vi "SPD.HV_Bias Test.vi"(5 "Graph":refnum<vi>, 7 "Progress":refnum<vi>, 8 "Error In":errorcluster, 11 "SPD.Stand Ctrl in":T1 {"spdDeviceSession"."hidSPD.Sturtup Values"."HV_bias" format="%#_6p, V"; "spdDeviceSession"."hidSPD.Sturtup Values"."TSet" format="%#_6p, DegC"; "spdDeviceSession"."hidSPD.Controller"."HV_bias" format="%#_6p, V"; "spdDeviceSession"."hidSPD.Controller"."TSet" format="%#_6p, DegC"}) -> (0 "Error Out":errorcluster, 1 "pass":bool, 3 "SPD.Stand Ctrl out":T1 {"spdDeviceSession"."hidSPD.Sturtup Values"."HV_bias" format="%#_6p, V"; "spdDeviceSession"."hidSPD.Sturtup Values"."TSet" format="%#_6p, DegC"; "spdDeviceSession"."hidSPD.Controller"."HV_bias" format="%#_6p, V"; "spdDeviceSession"."hidSPD.Controller"."TSet" format="%#_6p, DegC"})   [LabVIEW 2018]
uses:
  typedefs/SPD.Stand Ctrl.ctl
  Instruments/SPD HID Interface/hidSPDLibForLabView/LibVIs/hidSPD Controls/hidSPD Device Session.ctl
  Instruments/SPD HID Interface/hidSPDLibForLabView/LibVIs/hidSPD Controls/hidSPD Controller.ctl
  Instruments/SPD HID Interface/hidSPDLibForLabView/LibVIs/hidSPD Controls/hidSPD SPD Type.ctl
  Instruments/KC705 DevBoard/typedefs/DevB.Session.ctl
  Instruments/KeySight 53230A/typedefs/FreqC.Session.ctl
  Instruments/KeySight 8164B/KeySight 8164B LAN InstrLib/typedefs/KeySight 8164B control.ctl
  Instruments/LeCroy SDA830/typedefs/LeCroy.Session.ctl
  typedefs/SPD.Events.ctl
  ConfigFile/SPD.Config File ctrl.ctl
  <vilib>/Utility/config.llb/Config Data RefNum.ctl
  typedefs/SPD.Meas Result.ctl
  typedefs/SPD.Queues.ctl
  typedefs/SPD.Stand state.ctl
  SubVIs/Min_Max.ctl
  SubTests/01_HV_Bias Test/SPD.HV_Bias Test Limits.vi
  SubVIs/comparison mode.ctl
  Instruments/KeySight 8164B/KeySight 8164B LAN InstrLib.lvlib
  <vilib>/Utility/config.llb/NI_LVConfig.lvlib
  Instruments/SPD HID Interface/hidSPDLibForLabView/hidSPDLibForLabView.lvlib
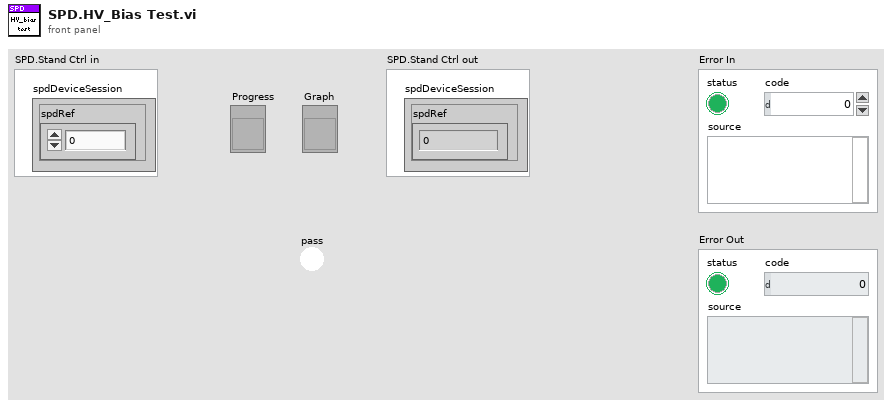
[diagram p1: front panel]
types:
  T1 = typedef "SPD.Stand Ctrl.ctl" = cluster{"spdDeviceSession":T2, "DevBSession":T5, "FreqCSession":T6, "8164BSession":T7, "LeCroySession":T8, "Events":T9, "configFile":T10, "SPD.Result":T12, "SPD.Queues":T13, "Console":refnum<vi>}
  T2 = typedef "hidSPDLibForLabView.lvlib/hidSPD Device Session.ctl" = cluster{"spdRef":u64, "connected":bool, "spdName":string, "hidSPD.Controller":T3, "hidSPD.Sturtup Values":T3, "SPD Type":T4}
  T3 = typedef "hidSPDLibForLabView.lvlib/hidSPD Controller.ctl" = cluster{"TSet":sgl, "HV_bias":sgl, "DDS_stb_code":u16}
  T4 = typedef "hidSPDLibForLabView.lvlib/hidSPD SPD Type.ctl" = enum16{"Free Run", "Gate"}
  T5 = typedef "DevB.Session.ctl" = cluster{"DevBRef":refnum<visa-resource-name>, "connected":bool}
  T6 = typedef "FreqC.Session.ctl" = cluster{"FreqCRef":refnum<visa-resource-name>, "timeout":dbl, "Gate":dbl, "connected":bool}
  T7 = typedef "KeySight 8164B LAN InstrLib.lvlib/KeySight 8164B control.ctl" = cluster{"Connection ID":refnum<k5>, "Connected":bool, "Info":string, "Slots Info":string[]}
  T8 = typedef "LeCroy.Session.ctl" = cluster{"LeCroySession":refnum<visa-resource-name>, "connected":bool}
  T9 = typedef "SPD.Events.ctl" = cluster{"DCRTest":refnum<user-event>, "Stop":refnum<user-event>}
  T10 = typedef "SPD.Config File ctrl.ctl" = cluster{"configFile ref":T11, "configFile path":path, "equipmentFile ref":T11}
  T11 = typedef "NI_LVConfig.lvlib/Config Data RefNum.ctl" = refnum<k1>
  T12 = typedef "SPD.Meas Result.ctl" = cluster{"HV_Bias":dbl[][][], "Stb_code":dbl[], "Temprature":dbl[], "Data":dbl[][][][], "DateTime":string}
  T13 = typedef "SPD.Queues.ctl" = cluster{"state queue":refnum<queue>}
  T14 = typedef "comparison mode.ctl" = enum16{"in range", "bigger then min", "bigger then max", "less then min", "less then max"}
  T15 = typedef "SPD.HV_Bias Test Limits.vi" = cluster{"start value":dbl, "stop value":dbl, "step":dbl, "gate":dbl, "num of tests":dbl, "range":T16, "comparison mode":T14}
  T16 = typedef "Min_Max.ctl" = cluster{"min":dbl, "max":dbl}
  T17 = typedef "SPD.HV_Bias Test Params.vi" = cluster{"FS":i32, "TS":i32, "Step_Quick":dbl, "Stop_Quick":dbl, "Start_Quick":dbl, "Gate_Quick":dbl, "Step_Precise":dbl, "Gate_Precise":dbl, "max":dbl, "min":dbl}
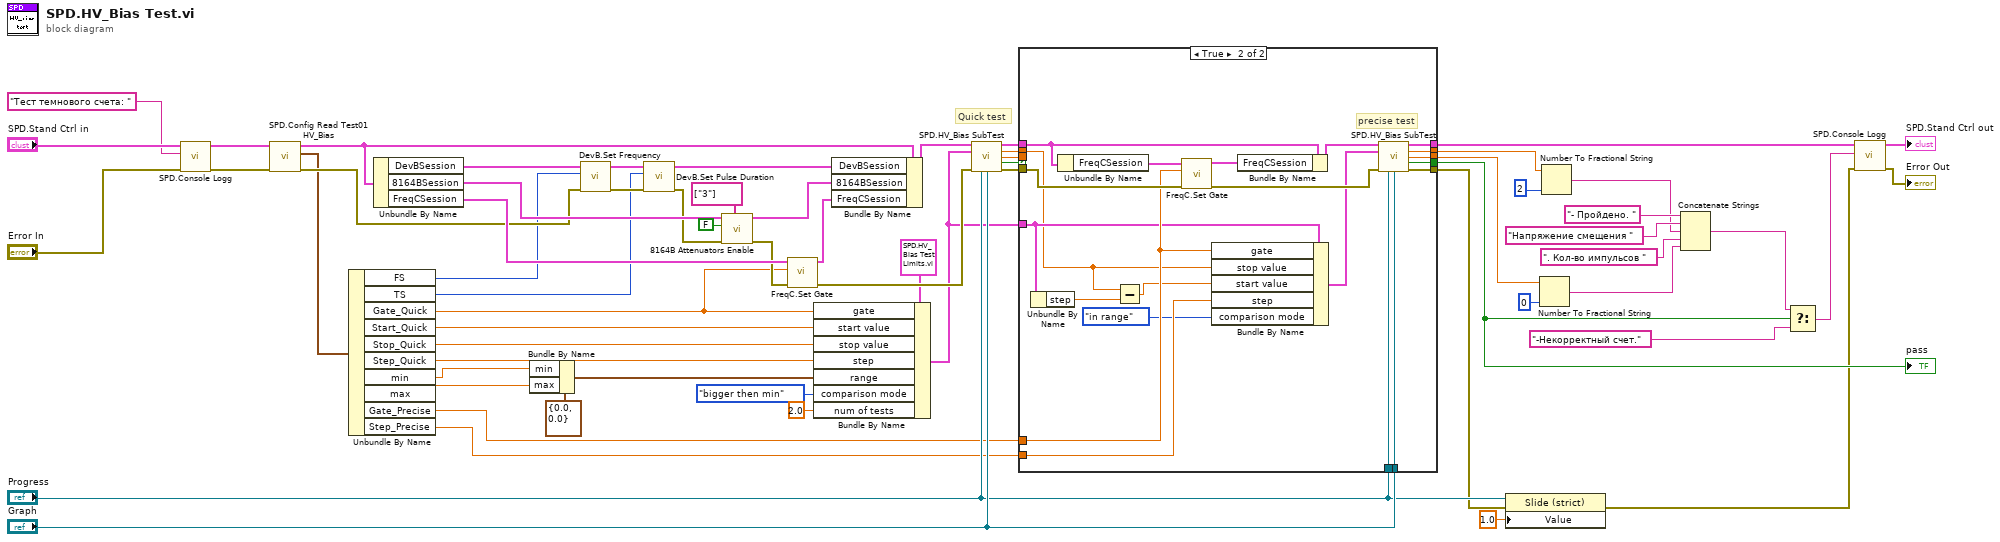
[diagram p0: block diagram]
diagram:
  # "Quick test"
  n1 = call "SPD.Console Logg.vi"("Error In"="Error In", "console Log"="Тест темнового счета: ", "SPD.Stand Ctrl in"="SPD.Stand Ctrl in") -> ("Error Out"=w7:errorcluster, "SPD.Stand Ctrl out"=w9:T1)  [unwired: 7 in]
  n2 = call "SPD.Config Read Test01 HV_Bias.vi"("Error In"=w7, "SPD.Stand Ctrl in"=w9) -> ("Error Out"=w41:errorcluster, "HV_TestParams"=w38:T17, "SPD.Stand Ctrl out"=w42:T1)  [unwired: 7 in]
  n3 = Unbundle By Name(w38) -> ("FS"=w37:i32, "TS"=w36:i32, "Gate_Quick"=w17:dbl, "Start_Quick"=w20:dbl, "Stop_Quick"=w19:dbl, "Step_Quick"=w18:dbl, "min"=w34:dbl, "max"=w33:dbl, "Gate_Precise"=w14:dbl, "Step_Precise"=w11:dbl)
  n4 = Unbundle By Name(w42) -> ("DevBSession"=w46:T5, "8164BSession"=w61:T7, "FreqCSession"=w60:T6)
  n5 = Bundle By Name(cluster=T16 {"min"=0.0, "max"=0.0} ("minMax"), "min"=w34, "max"=w33) -> (w16:T16)
  n6 = call "DevB.Set Frequency.vi"("error in (no error)"=w41, "Frequency"=w37, "DevB Session in"=w46) -> ("error out"=w47:errorcluster, "DevB Session out"=w48:T5)  [unwired: 7 in]
  n7 = call "DevB.Set Pulse Duration.vi"("error in (no error)"=w47, "Pulse Duration"=w36, "DevB Session in"=w48) -> ("error out"=w44:errorcluster, "DevB Session out"=w45:T5)  [unwired: 7 in]
  n8 = call "8164B Attenuators Enable.vi"("Slots"=string[] ["3"], "error in"=w44, "Enable"=FALSE, "KeySight 8164B control in"=w61) -> ("error out"=w59:errorcluster, "KeySight 8164B control out"=w58:T7)  [unwired: 6 in]
  n9 = call "FreqC.Set Gate.vi"("error In"=w59, "Gate, sec"=w17, "FreqC Session in"=w60) -> ("error out"=w39:errorcluster, "FreqC Session out"=w57:T6)  [unwired: 7 in]
  n10 = Bundle By Name(cluster=T15 {"start value"=0.0, "stop value"=0.0, "step"=0.0, "gate"=0.0, "num of tests"=0.0, "range"={"min"=0.0, "max"=0.0}, "comparison mode"=enum."in range"} ("SPD.HV_bias Test Limits"), "gate"=w17, "start value"=w20, "stop value"=w19, "step"=w18, "range"=w16, "comparison mode"=comparison_mode."bigger then min", "num of tests"=2.0) -> (w13:T15)
  n11 = Bundle By Name(cluster=w42, "DevBSession"=w45, "8164BSession"=w58, "FreqCSession"=w57) -> (w40:T1)
  n12 = call "SPD.HV_Bias SubTest.vi"("SPD.Stand Ctrl in"=w40, "SPD.HV_bias Test Limits"=w13, "Error In"=w39, "Progress"="Progress", "Graph"="Graph") -> ("SPD.Stand Ctrl out"=w31:T1, "last HV_bias"=w29:dbl, "Clicks Count"=w22:dbl, "result"=w24:bool, "Error Out"=w30:errorcluster)  [unwired: 6 in]
  n13 = case shown="True" w24 {
    selector: w24 -> [w68 _]
    tunnel: "Graph" -> [_ w90]
    tunnel: w14 -> [_ w76]
    tunnel: w31 -> [w69 w88]
    tunnel: w30 -> [w67 w86]
    tunnel: w29 -> [w66 w73]
    tunnel: "Progress" -> [_ w84]
    tunnel: [w67 w83] -> w27
    tunnel: [w69 w81] -> w5
    tunnel: [w66 w80] -> w26
    tunnel: [w65 w79] -> w25
    tunnel: [w68 w78] -> w23
    tunnel: w22 -> [w65 _]
    tunnel: w13 -> [_ w75]
    tunnel: w11 -> [_ w71]
    frame False {
    }
    frame True {
      # "precise test"
      n14 = Unbundle By Name(w75) -> ("step"=w74:dbl)
      n15 = Unbundle By Name(w88) -> ("FreqCSession"=w89:T6)
      n16 = Subtract(x=w73, y=w74) -> (x-y=w72:dbl)
      n17 = call "FreqC.Set Gate.vi"("error In"=w86, "Gate, sec"=w76, "FreqC Session in"=w89) -> ("error out"=w82:errorcluster, "FreqC Session out"=w87:T6)  [unwired: 7 in]
      n18 = Bundle By Name(cluster=w75, "gate"=w76, "stop value"=w73, "start value"=w72, "step"=w71, "comparison mode"=comparison_mode."in range" ("Comparison Mode")) -> (w77:T15)
      n19 = Bundle By Name(cluster=w88, "FreqCSession"=w87) -> (w85:T1)
      n20 = call "SPD.HV_Bias SubTest.vi"("SPD.Stand Ctrl in"=w85, "SPD.HV_bias Test Limits"=w77, "Error In"=w82, "Progress"=w84, "Graph"=w90) -> ("SPD.Stand Ctrl out"=w81:T1, "last HV_bias"=w80:dbl, "Clicks Count"=w79:dbl, "result"=w78:bool, "Error Out"=w83:errorcluster)  [unwired: 6 in]
    }
  }
  "pass" <- w23
  n21 = property class="Slide (strict)"(reference="Progress", error in=w27, "Value"=1.0) -> (error out=w2:errorcluster)  [unwired: 1 out]
  n22 = Number To Fractional String(number=w25, precision (6)=i16 0) -> (F-format string=w50:string)  [unwired: 2 in]
  n23 = Number To Fractional String(number=w26, precision (6)=i16 2) -> (F-format string=w53:string)  [unwired: 2 in]
  n24 = Concatenate Strings("- Пройдено. " ("report"), "Напряжение смещения " ("report"), w53, ". Кол-во импульсов " ("report"), w50) -> (w56:string)
  n25 = Select(t=w56, s=w23, f="-Некорректный счет.") -> (s? t:f=w3:string)
  n26 = call "SPD.Console Logg.vi"("Error In"=w2, "console Log"=w3, "SPD.Stand Ctrl in"=w5) -> ("Error Out"=→"Error Out":errorcluster, "SPD.Stand Ctrl out"=→"SPD.Stand Ctrl out":T1)  [unwired: 7 in]
